vi "Runtime.Async.vi"(10 "Parameters":variant, 11 "Process":refnum<class "Process.lvclass">) -> ()   [LabVIEW 2015, in "DMM-SWITCH-ScanList Engine.lvlib"]
uses:
  DMM-SWITCH-ScanList Engine.lvlib
  <vilib>/NI Veristand/Custom Device API/Custom Device Item Ref.ctl
  <vilib>/addons/Inline Async API/_VS Inline Async API/Process/Process.lvclass
  Shared/Compiled.Settings
  TypeDefs/DMM-Switch Configuration.ctl
  <instrlib>/niDMM/nidmm.llb/niDMM Function.ctl
  <instrlib>/niDMM/nidmm.llb/niDMM Resolution in Digits.ctl
  <instrlib>/niSwitch/niSwitch.LLB/niSwitch Topologies.ctl
  <instrlib>/niSwitch/niSwitch.LLB/niSwitch Trigger Input.ctl
  <instrlib>/niSwitch/niSwitch.LLB/niSwitch Scan Advanced Output.ctl
  <instrlib>/niDMM/nidmm.llb/niDMM Measurement Complete.ctl
  <instrlib>/niDMM/nidmm.llb/niDMM Trigger.ctl
  <vilib>/addons/Inline Async API/_VS Inline Async API/Process/Process.lvclass/Process.ctl
  <vilib>/addons/Inline Async API/_Data Access Engine/Access Type Classes/ReadWrite/ReadWrite.lvclass/ReadWrite.ctl
  <vilib>/addons/Inline Async API/_Data Access Engine/Access Type Classes/Write/Write.lvclass/Write.ctl
  <vilib>/addons/Inline Async API/_Data Access Engine/Data Access Engine/Methods/Write.Data.vi
  <vilib>/addons/Inline Async API/_Data Access Engine/Data Access Engine/Methods/ReadWrite.Data.vi
  <vilib>/addons/Inline Async API/_VS Inline Async API/Process/Data Member Access/Read Data Access.vi
  <vilib>/addons/Inline Async API/_Data Access Engine/Access Type Classes/Write/Write.ProcessData.vi
  <vilib>/addons/Inline Async API/_VS Inline Async API/Error Handling Process/SubVIs/Error.ConvertArray.vi
  <vilib>/addons/Inline Async API/_Data Access Engine/Access Type Classes/ReadWrite/ReadWrite.ProcessData.vi
  <vilib>/addons/Inline Async API/_Data Access Engine/Data Access Engine/Methods/Write.Lookup.vi
  <vilib>/addons/Inline Async API/_Data Access Engine/Data Access Engine/Methods/ReadWrite.Lookup.vi
  <vilib>/NI Veristand/Custom Device Tools/Custom Device Utility Library/NI VeriStand - Search for Item by Name.vi
  <vilib>/addons/Inline Async API/_Data Access Engine/Data Access Engine/Data Access Engine.lvclass
  <vilib>/NI Veristand/Custom Device Tools/Custom Device Utility Library/Custom Device Utility Library.lvlib
  <vilib>/NI Veristand/Custom Device API/Custom Device API.lvlib
  Shared/DMM-SWITCH-ScanList Shared.lvlib
panel:
  in  "Device Reference":T1 format="%.0x"
  in  "Device Clock":string
  # "Custom Device Template\nv1.0"
  # "Use this template as a starting point for creating a custom device code module. The input controls shown here are specially named controls that the system will use to provide the device loop with data. The controls are not required for the device loop to run. For instance, if the device doesn't produce any output data, then you don't need the Device Outputs FIFO control. If you do use these controls, however, they need to have these exact names to be functional."
  # "The optional status notifier element is used to notify the RT engine of the last state of the custom device, and to indicate the device has completed execution. If this control is not used, a default No Error value is returned to the system when the device finishes execution.\n\nNote: This error state is not checked until the system shuts down. Use an output status channel to send more immediate status values to the system."
  # "This optional input can be used to send the VeriStand Engine the final status of the custom device initalization process. If this control exists on the custom device front panel, the VeriStand Engine will wait for a status update before starting up. If the custom device reports an error, that will abort the execution of the current configuration in the VeriStand Engine.\n\nThis control can be deleted if the custom device does not need to send the initialization status update."
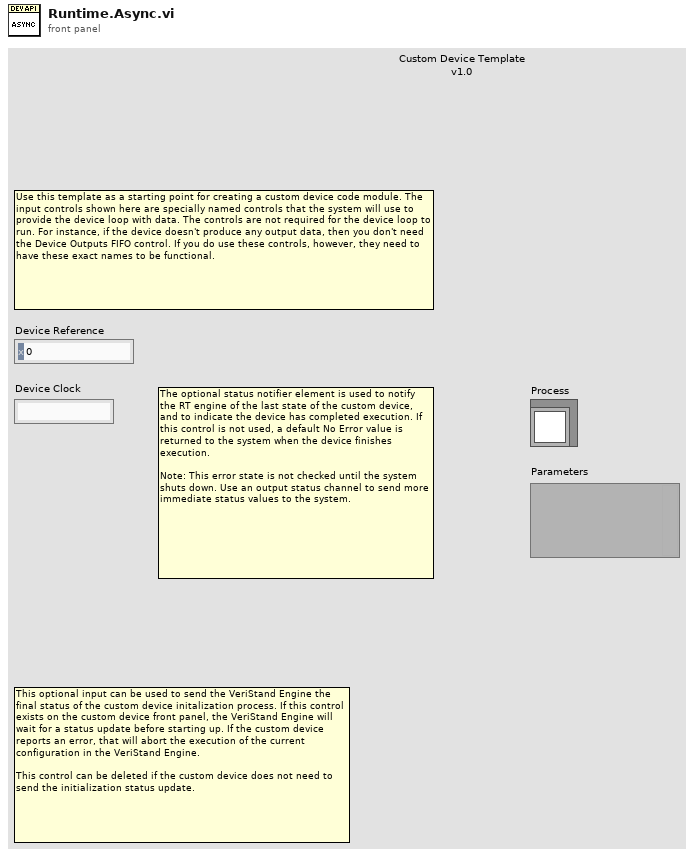
[diagram p1: front panel]
types:
  T1 = typedef "Custom Device API.lvlib/Custom Device Item Ref.ctl" = u64
  T2 = typedef "DMM-SWITCH-ScanList Shared.lvlib/Compiled.Settings" = cluster{"Name":string, "DMM-Switch Configuration":T3}
  T3 = typedef "DMM-SWITCH-ScanList Engine.lvlib/DMM-Switch Configuration.ctl" = cluster{"DMM Resource Name":string, "DMM Measurement":T4, "DMM Resolution in Digits":T5, "DMM Range [EU]":dbl, "Switch Resource Name":string, "Switch Topology":T6, "Switch Scan List":string, "Switch Trigger Source":T7, "Switch Scan Advanced Output":T8, "DMM Measurement Complete":T9, "DMM Trigger Source":T10, "# of Channels":u32, "Group CH Names - Configuration":string, "Group CH Names - Input Channels":string, "Group CH Names - Measurement Channels":string, "Group CH Names - Runtime Status":string}
  T4 = typedef "niDMM Function.ctl" = enum16{"DC Volts", "AC Volts", "DC Current", "AC Current", "2-wire Resistance", "4-wire Resistance", "Diode", "Frequency", "Period", "AC Volts DC Coupled", "Capacitance", "Inductance", "Temperature"}
  T5 = typedef "niDMM Resolution in Digits.ctl" = dbl
  T6 = typedef "niSwitch Topologies.ctl" = string
  T7 = typedef "niSwitch Trigger Input.ctl" = enum16{"Immediate", "External", "TTL0", "TTL1", "TTL2", "TTL3", "TTL4", "TTL5", "TTL6", "TTL7", "ECL0", "ECL1", "PXI Star", "Software Trigger Function", "Rear Connector", "Front Connector", "Rear Connector of Module 1", "Rear Connector of Module 2", "Rear Connector of Module 3", "Rear Connector of Module 4", "Rear Connector of Module 5", "Rear Connector of Module 6", "Rear Connector of Module 7", "Rear Connector of Module 8", "Rear Connector of Module 9", "Rear Connector of Module 10", "Rear Connector of Module 11", "Rear Connector of Module 12", "Front Connector of Module 1", "Front Connector of Module 2", "Front Connector of Module 3", "Front Connector of Module 4", "Front Connector of Module 5", "Front Connector of Module 6", "Front Connector of Module 7", "Front Connector of Module 8", "Front Connector of Module 9", "Front Connector of Module 10", "Front Connector of Module 11", "Front Connector of Module 12"}
  T8 = typedef "niSwitch Scan Advanced Output.ctl" = enum16{"None", "External", "TTL0", "TTL1", "TTL2", "TTL3", "TTL4", "TTL5", "TTL6", "TTL7", "ECL0", "ECL1", "PXI Star", "Rear Connector", "Front Connector", "Rear Connector Module 1", "Rear Connector Module 2", "Rear Connector Module 3", "Rear Connector Module 4", "Rear Connector Module 5", "Rear Connector Module 6", "Rear Connector Module 7", "Rear Connector Module 8", "Rear Connector Module 9", "Rear Connector Module 10", "Rear Connector Module 11", "Rear Connector Module 12", "Front Connector Module 1", "Front Connector Module 2", "Front Connector Module 3", "Front Connector Module 4", "Front Connector Module 5", "Front Connector Module 6", "Front Connector Module 7", "Front Connector Module 8", "Front Connector Module 9", "Front Connector Module 10", "Front Connector Module 11", "Front Connector Module 12"}
  T9 = typedef "niDMM Measurement Complete.ctl" = enum16{"None", "External", "TTL 0", "TTL 1", "TTL 2", "TTL 3", "TTL 4", "TTL 5", "TTL 6", "TTL 7", "LBR Trig 0"}
  T10 = typedef "niDMM Trigger.ctl" = enum16{"Immediate", "External", "TTL 0", "TTL 1", "TTL 2", "TTL 3", "TTL 4", "TTL 5", "TTL 6", "Software", "TTL 7", "PXI Star", "LBR Trig 1", "Aux Trig 1"}
  T11 = enum16{"Open or Create File", "Write Error", "Close File"}
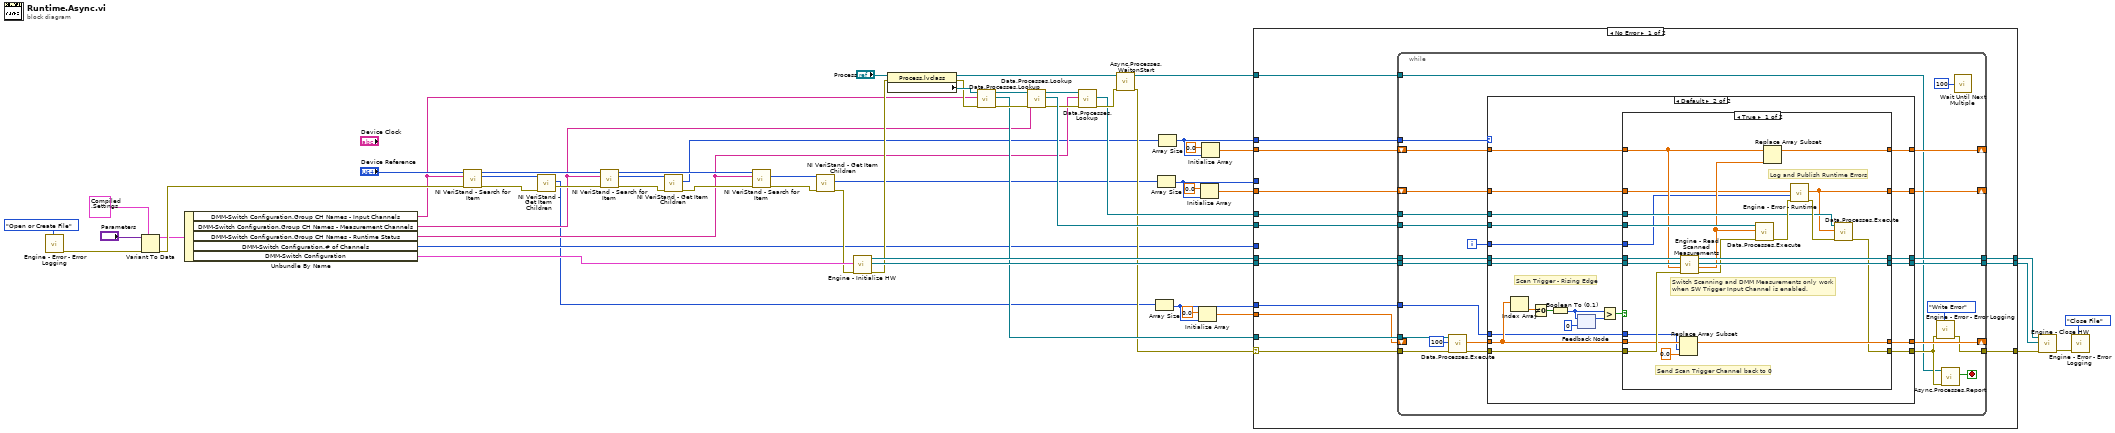
[diagram p0: block diagram]
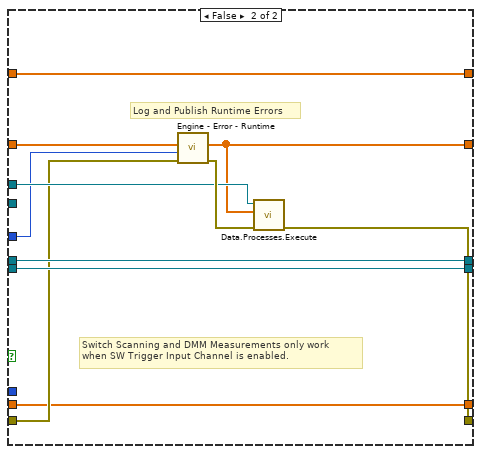
[diagram p3: hidden frame]
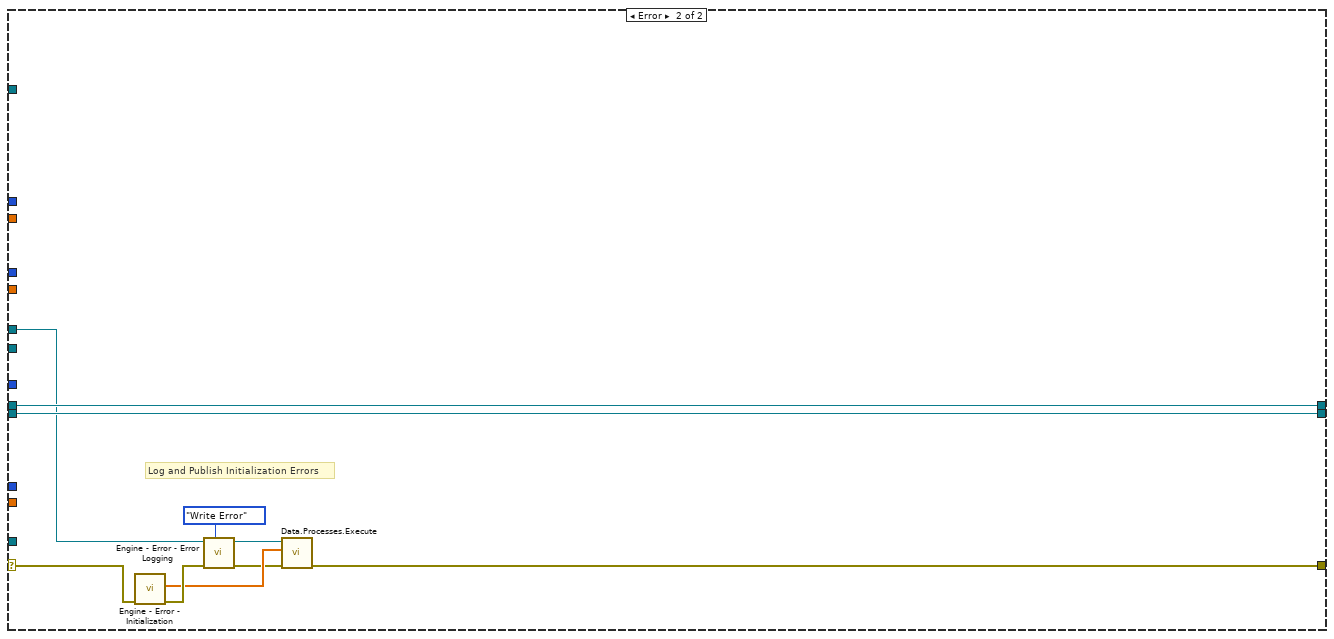
[diagram p4: hidden frame]
diagram:
  n1 = call "Engine - Error - Error Logging.vi"("Error Log FGV Cmd"=T11."Open or Create File") -> ("error out"=w20:errorcluster)  [unwired: 10 in]
  n2 = Variant To Data(error in=w20, type=T2 {"Name"="", "DMM-Switch Configuration"={"DMM Resource Name"="", "DMM Measurement"=enum."DC Volts", "DMM Resolution in Digits"=6.5, "DMM Range [EU]"=10.0, "Switch Resource Name"="", "Switch Topology"="2503/2-Wire 24x1 Mux", "Switch Scan List"="ab0->com0 & com0->ch0:2;", "Switch Trigger Source"=enum."TTL0", "Switch Scan Advanced Output"=enum."TTL1", "DMM Measurement Complete"=enum."TTL 0", "DMM Trigger Source"=enum."TTL 1", "# of Channels"=0, "Group CH Names - Configuration"="", "Group CH Names - Input Channels"="", "Group CH Names - Measurement Channels"="", "Group CH Names - Runtime Status"=""}} ("Parameters"), Variant="Parameters") -> (data=w21:T2, error out=w22:errorcluster)
  n3 = Unbundle By Name(w21) -> ("DMM-Switch Configuration.Group CH Names - Input Channels"=w15:string, "DMM-Switch Configuration.Group CH Names - Measurement Channels"=w14:string, "DMM-Switch Configuration.Group CH Names - Runtime Status"=w13:string, "DMM-Switch Configuration.# of Channels"=w16:u32, "DMM-Switch Configuration"=w43:T3)
  n4 = call-poly <vilib>:"NI VeriStand - Search for Item.vi"("error in"=w22, "Item Name"=w15, "Section Ref in"="Device Reference") -> ("error out"=w37:errorcluster, "Item Ref"=w35:T1, "Section Ref out"=w30:T1)  [unwired: 5 in, 1 out]
  n5 = call <vilib>:"NI VeriStand - Get Item Children.vi"("error in (no error)"=w37, "Item Ref in"=w35) -> ("error out"=w31:errorcluster, "Child Refs"=w3:T1[])  [unwired: 6 in, 2 out]
  n6 = call-poly <vilib>:"NI VeriStand - Search for Item.vi"("error in"=w31, "Item Name"=w14, "Section Ref in"=w30) -> ("error out"=w32:errorcluster, "Item Ref"=w33:T1, "Section Ref out"=w27:T1)  [unwired: 5 in, 1 out]
  n7 = call <vilib>:"NI VeriStand - Get Item Children.vi"("error in (no error)"=w32, "Item Ref in"=w33) -> ("error out"=w26:errorcluster, "Child Refs"=w11:T1[])  [unwired: 6 in, 2 out]
  n8 = call-poly <vilib>:"NI VeriStand - Search for Item.vi"("error in"=w26, "Item Name"=w13, "Section Ref in"=w27) -> ("error out"=w29:errorcluster, "Item Ref"=w28:T1)  [unwired: 5 in, 2 out]
  n9 = call <vilib>:"NI VeriStand - Get Item Children.vi"("error in (no error)"=w29, "Item Ref in"=w28) -> ("error out"=w25:errorcluster, "Child Refs"=w7:T1[])  [unwired: 6 in, 2 out]
  n10 = call "Engine - Initialize HW.vi"("error in (no error)"=w25, "DMM-Switch Configuration"=w43) -> ("error out"=w19:errorcluster, "DMM Ref Out"=w56:refnum<k15>, "Switch Ref Out"=w57:refnum<k15>)  [unwired: 7 in]
  n11 = property class="Process.lvclass"(reference="Process", error in=w19) -> (reference out=w46:refnum<class "Process.lvclass">, error out=w18:errorcluster, "Data Member Access:Data Access"=w45:refnum<class "Data Access Engine.lvclass">)
  n12 = call-poly <vilib>:"Data.Processes.Lookup.vi"("error in (no error)"=w18, "Name"=w15, "Data Access API in"=w45) -> ("error out"=w49:errorcluster, "Ref"=w42:refnum<data-value>, "Data Access API out"=w48:refnum<class "Data Access Engine.lvclass">)  [unwired: 6 in]
  n13 = call-poly <vilib>:"Data.Processes.Lookup.vi"("error in (no error)"=w49, "Name"=w14, "Data Access API in"=w48) -> ("error out"=w39:errorcluster, "Ref"=w41:refnum<data-value>, "Data Access API out"=w40:refnum<class "Data Access Engine.lvclass">)  [unwired: 6 in]
  n14 = call-poly <vilib>:"Data.Processes.Lookup.vi"("error in (no error)"=w39, "Name"=w13, "Data Access API in"=w40) -> ("error out"=w38:errorcluster, "Ref"=w34:refnum<data-value>)  [unwired: 6 in, 1 out]
  n15 = call <vilib>:"Async.Processes.WaitonStart.vi"("error in (no error)"=w38, "Process"=w46) -> ("error out"=w17:errorcluster, "Process out"=w44:refnum<class "Process.lvclass">)  [unwired: 7 in, 1 out]
  n16 = Array Size(array=w3) -> (size(s)=w2:i32)
  n17 = Array Size(array=w7) -> (size(s)=w5:i32)
  n18 = Array Size(array=w11) -> (size(s)=w10:i32)
  n19 = Initialize Array(0.0 ("element"), w2) -> (w1:dbl[])
  n20 = Initialize Array(0.0 ("element"), w5) -> (w6:dbl[])
  n21 = Initialize Array(0.0 ("element"), w10) -> (w9:dbl[])
  n22 = case shown="No Error" w17 {
    selector: w17 -> [w69 w166]
    tunnel: w42 -> [w72 _]
    tunnel: w2 -> [w58 _]
    tunnel: w10 -> [w62 _]
    tunnel: w57 -> [w71 w165]
    tunnel: w56 -> [w70 w164]
    tunnel: [w68 w158] -> w55
    tunnel: [w67 w165] -> w54
    tunnel: [w66 w164] -> w53
    tunnel: w41 -> [w65 _]
    tunnel: w44 -> [w64 _]
    tunnel: w34 -> [w63 w160]
    tunnel: w5 -> [_ _]
    tunnel: w16 -> [_ _]
    tunnel: w9 -> [w61 _]
    tunnel: w6 -> [w60 _]
    tunnel: w1 -> [w59 _]
    frame No Error {
      n23 = while {
        shift-right: [w97] -> _
        shift-left: w59 -> [_]
        shift-right: [w95] -> _
        shift-left: w61 -> [w96]
        tunnel: w62 -> [w73]
        tunnel: w65 -> [w94]
        tunnel: w72 -> [w81]
        tunnel: w58 -> [w79]
        tunnel: w70 -> [w93]
        tunnel: w71 -> [w92]
        tunnel: [w91] -> w67
        tunnel: [w90] -> w66
        tunnel: w64 -> [w82]
        tunnel: w63 -> [w78]
        shift-right: [w76] -> _
        shift-left: w60 -> [w77]
        tunnel: w69 -> [w89]
        tunnel: [w85] -> w68
        i -> [w75]
        stop <- w83 stop-if-true
        n24 = call-poly <vilib>:"Data.Processes.Execute.vi"("error in (no error)"=w89, "timeout ms"=100, "Ref"=w81) -> ("error out"=w87:errorcluster, "Data"=w88:dbl[])  [unwired: 6 in, 1 out]
        n25 = case shown="Default" w73 {
          tunnel: w94 -> [_ w114]
          tunnel: w96 -> [w103 w120]
          tunnel: w88 -> [w102 w117]
          tunnel: w87 -> [w101 w123]
          tunnel: [w101 w108] -> w84
          tunnel: [w103 w119] -> w95
          tunnel: [w102 w116] -> w97
          tunnel: w93 -> [w99 w125]
          tunnel: w92 -> [w100 w124]
          tunnel: [w100 w122] -> w91
          tunnel: [w99 w121] -> w90
          tunnel: w75 -> [_ w115]
          tunnel: w79 -> [_ w107]
          tunnel: w78 -> [_ w106]
          tunnel: w77 -> [w98 w105]
          tunnel: [w98 w104] -> w76
          frame 0 {
            # "No outputs to write to system. The Device Outputs FIFO is never created in this case, so don't write to it."
          }
          frame Default {
            # "Scan Trigger - Rising Edge"
            n26 = Index Array(array=w117) -> (element=w118:dbl)  [unwired: 1 in]
            n27 = Not Equal To 0?(x=w118) -> (x != 0?=w113:bool)
            n28 = Boolean To (0,1)(Boolean=w113) -> (0, 1=w112:i16)
            n29 = feedback-in #1(w112) -> ()
            n30 = feedback #1(i16 0) -> (w111:i16)
            n31 = Greater?(x=w112, y=w111) -> (0:w109:bool)
            n32 = case shown="True" w109 {
              tunnel: w125 -> [w146 w150]
              tunnel: w124 -> [w145 w151]
              tunnel: w123 -> [w144 w149]
              tunnel: [w143 w151] -> w122
              tunnel: [w142 w150] -> w121
              tunnel: w120 -> [w131 w152]
              tunnel: [w129 w152] -> w119
              tunnel: [w133 w156] -> w108
              tunnel: w117 -> [w141 w148]
              tunnel: [w140 w148] -> w116
              tunnel: w115 -> [w126 w147]
              tunnel: w114 -> [w137 _]
              tunnel: w107 -> [w138 _]
              tunnel: w106 -> [w132 w155]
              tunnel: w105 -> [w128 w154]
              tunnel: [w127 w153] -> w104
              frame True {
                # "Log and Publish Runtime Errors"
                # "Send Scan Trigger Channel back to 0"
                # "Switch Scanning and DMM Measurements only work\nwhen SW Trigger Input Channel is enabled."
                n33 = Replace Array Subset(array=w141, new element=0.0 ("new element/subarray"), index=w138) -> (w140:dbl[])
                n34 = call "Engine - Read Scanned Measurements.vi"("error in (no error)"=w144, "Output Channels Array In"=w131, "DMM Ref In"=w146, "Switch Ref In"=w145) -> ("error out"=w136:errorcluster, "Output Channels Array Out"=w130:dbl[], "DMM Ref Out"=w142:refnum<k15>, "Switch Ref Out"=w143:refnum<k15>)  [unwired: 4 in]
                n35 = call-poly <vilib>:"Data.Processes.Execute.vi"("error in (no error)"=w136, "Values"=w130, "Ref"=w137) -> ("error out"=w135:errorcluster)  [unwired: 8 in]
                n36 = Replace Array Subset(array=w131, new element=w130) -> (w129:dbl[])  [unwired: 1 in]
                n37 = call "Engine - Error - Runtime.vi"("error in (no error)"=w135, "Iteration"=w126, "Runtime Status Channels In"=w128) -> ("error out"=w134:errorcluster, "Runtime Status Channels In"=w127:dbl[])  [unwired: 7 in]
                n38 = call-poly <vilib>:"Data.Processes.Execute.vi"("error in (no error)"=w134, "Values"=w127, "Ref"=w132) -> ("error out"=w133:errorcluster)  [unwired: 8 in]
              }
              frame False {
                # "Log and Publish Runtime Errors"
                # "Switch Scanning and DMM Measurements only work\nwhen SW Trigger Input Channel is enabled."
                n39 = call "Engine - Error - Runtime.vi"("error in (no error)"=w149, "Iteration"=w147, "Runtime Status Channels In"=w154) -> ("error out"=w157:errorcluster, "Runtime Status Channels In"=w153:dbl[])  [unwired: 7 in]
                n40 = call-poly <vilib>:"Data.Processes.Execute.vi"("error in (no error)"=w157, "Values"=w153, "Ref"=w155) -> ("error out"=w156:errorcluster)  [unwired: 8 in]
              }
            }
          }
        }
        n41 = call "Engine - Error - Error Logging.vi"("Error Log FGV Cmd"=T11."Write Error", "error in (no error)"=w84) -> ("error out"=w85:errorcluster)  [unwired: 9 in]
        n42 = call <vilib>:"Async.Processes.Report.vi"("Error"=w84, "Process in"=w82) -> ("Stop"=w83:bool)  [unwired: 8 in, 1 out]
        n43 = call "Wait Until Next Multiple"("Count(mSec)"=u32 100 ("milliseconds to wait")) -> ()  [unwired: 1 out]
      }
    }
    frame Error {
      # "Log and Publish Initialization Errors"
      n44 = call "Engine - Error - Initialization.vi"("error in (no error)"=w166) -> ("error out"=w162:errorcluster, "Runtime Status Channels Out"=w161:dbl[])  [unwired: 9 in]
      n45 = call "Engine - Error - Error Logging.vi"("Error Log FGV Cmd"=T11."Write Error", "error in (no error)"=w162) -> ("error out"=w159:errorcluster)  [unwired: 9 in]
      n46 = call-poly <vilib>:"Data.Processes.Execute.vi"("error in (no error)"=w159, "Values"=w161, "Ref"=w160) -> ("error out"=w158:errorcluster)  [unwired: 8 in]
    }
  }
  n47 = call "Engine - Close HW.vi"("error in (no error)"=w55, "DMM Ref In"=w53, "SWITCH Ref In"=w54) -> ("error out"=w50:errorcluster)  [unwired: 8 in]
  n48 = call "Engine - Error - Error Logging.vi"("Error Log FGV Cmd"=T11."Close File", "error in (no error)"=w50) -> ()  [unwired: 9 in, 1 out]
